vi "getText.vi"(0 "reference":refnum<class "NoteNode.lvclass">, 5 "error in (no error)":errorcluster) -> (14 "reference out":refnum<class "NoteNode.lvclass">, 15 "text":refnum<class "MultiLineString.lvclass">, 19 "error out":errorcluster)   [LabVIEW 2014, in "NoteNode.lvclass"]
doc: "public MultiLineString getText()"
uses:
  <resource>/Framework/Providers/Open_GDS/UML/NoteNode_class/NoteNode.lvclass
  <resource>/Framework/Providers/Open_GDS/UML/MultiLineString_class/MultiLineString.lvclass
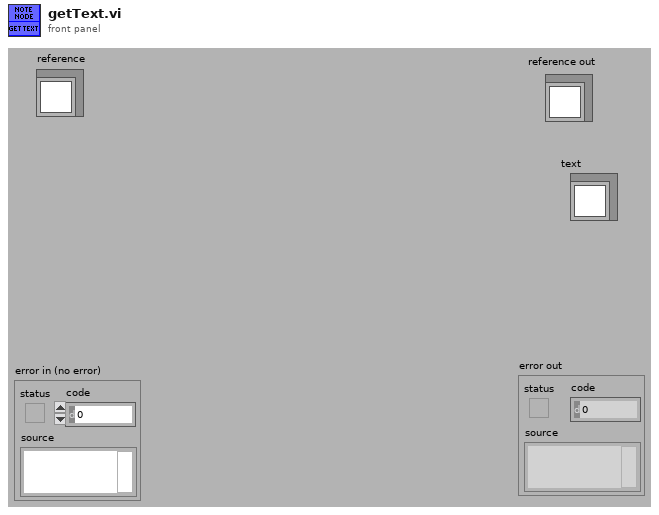
[diagram p1: front panel]
types:
  T1 = typedef "NoteNode.lvclass/ObjectAttributes.ctl" = cluster{"DEFAULT_WIDTH":i32, "DEFAULT_HEIGHT":i32, "DEFAULT_COLOR":u32, "FOLD_X":i32, "FOLD_Y":i32, "color":u32, "text":refnum<class "MultiLineString.lvclass">, "pointNodes":refnum<class "AbstractNode.lvclass">[]}
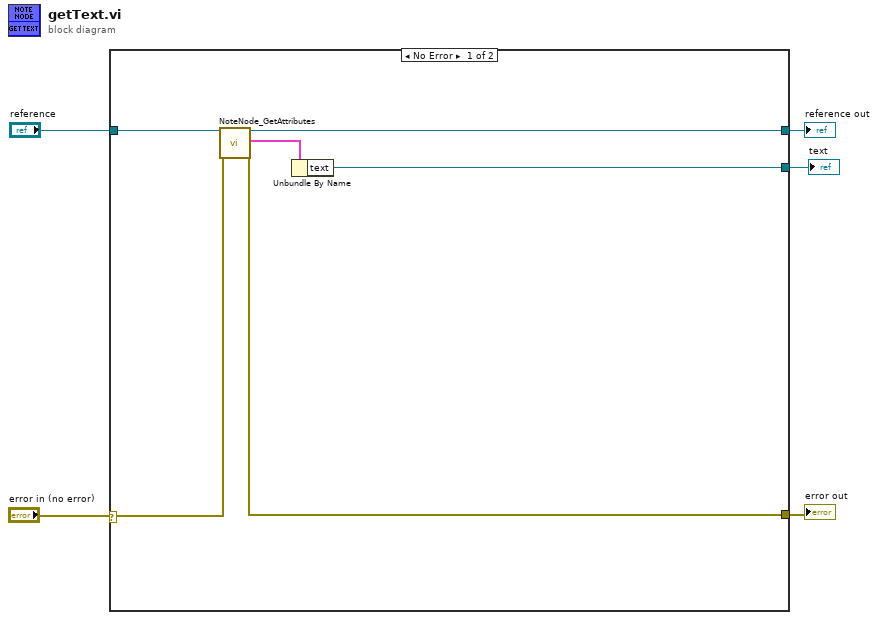
[diagram p0: block diagram]
diagram:
  n1 = case shown="No Error" "error in (no error)" {
    selector: "error in (no error)" -> [w8 w12]
    tunnel: "reference" -> [w11 w13]
    tunnel: [w10 w12] -> w4
    tunnel: [w9 w13] -> w3
    tunnel: [w7 _] -> w1
    frame No Error {
      n2 = call <resource>:"NoteNode_GetAttributes.vi"("reference in"=w11, "error in (no error)"=w8) -> ("reference out"=w9:refnum<class "NoteNode.lvclass">, "Data"=w6:T1, "error out"=w10:errorcluster)  [unwired: 1 in, 14 out]
      n3 = Unbundle By Name(w6) -> ("text"=w7:refnum<class "MultiLineString.lvclass">)
    }
    frame Error {
    }
  }
  "reference out" <- w3
  "error out" <- w4
  "text" <- w1
